vi "fix dynamic discovery.vi"(8 "error in":errorcluster, 10 "DecideProjectFeatures in":refnum<class "TagBusConfigurablePluginDecideFeatures.lvclass">, 11 "User Project in":refnum<vi>) -> (0 "error out":errorcluster, 3 "User Project out":refnum<vi>)   [LabVIEW 2013, in "TagBusConfigurablePluginDecideFeatures.lvclass"]
uses:
  TagBusConfigurablePluginDecideFeatures.lvclass
  TagBusConfigurablePluginDecideFeatures.lvclass/TagBusConfigurablePluginDecideFeatures.ctl
  Read discovers channels dynamically.vi
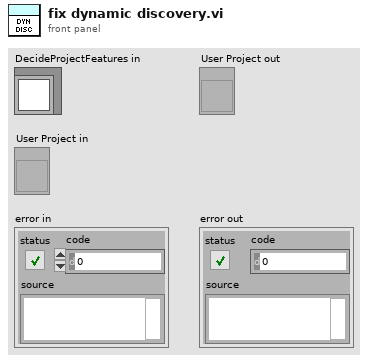
[diagram p1: front panel]
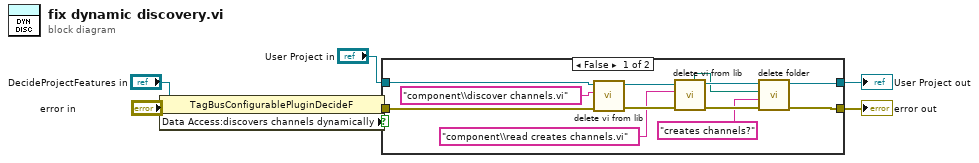
[diagram p0: block diagram]
diagram:
  n1 = property class="TagBusConfigurablePluginDecideF"(reference="DecideProjectFeatures in", error in="error in") -> (error out=w4:errorcluster, "Data Access:discovers channels dynamically"=w3:bool)  [unwired: 1 out]
  n2 = case shown="False" w3 {
    tunnel: "User Project in" -> [w19 w21]
    tunnel: w4 -> [w18 w20]
    tunnel: [w12 w21] -> w2
    tunnel: [w11 w20] -> w1
    frame False {
      n3 = call "delete vi from lib.vi"("error in"=w18, "relative path"="component\\discover channels.vi", "Project in"=w19) -> ("error out"=w15:errorcluster, "Project out"=w16:refnum<vi>)  [unwired: 6 in, 1 out]
      n4 = call "delete vi from lib.vi"("error in"=w15, "relative path"="component\\read creates channels.vi", "Project in"=w16) -> ("error out"=w10:errorcluster, "Project out"=w13:refnum<vi>, "lib path"=w9:path)  [unwired: 6 in]
      n5 = call "delete folder.vi"("error in"=w10, "folder"="creates channels?", "lib path"=w9, "Project in"=w13) -> ("error out"=w11:errorcluster, "Project out"=w12:refnum<vi>)  [unwired: 6 in]
    }
    frame True {
    }
  }
  "error out" <- w1
  "User Project out" <- w2
